vi "startAD.vi"() -> ()   [LabVIEW 2018]
uses:
  main/PCI8552B_32.dll
panel:
  out "待读取数据长度":i32
  out "波形图":dbl[][](graph)
  out "Data":dbl[][](array[numeric])
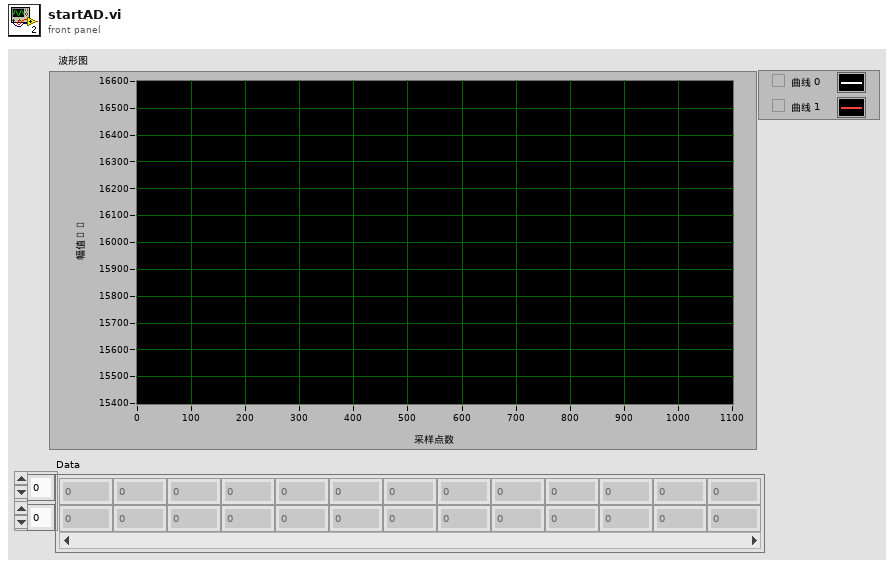
[diagram p1: front panel]
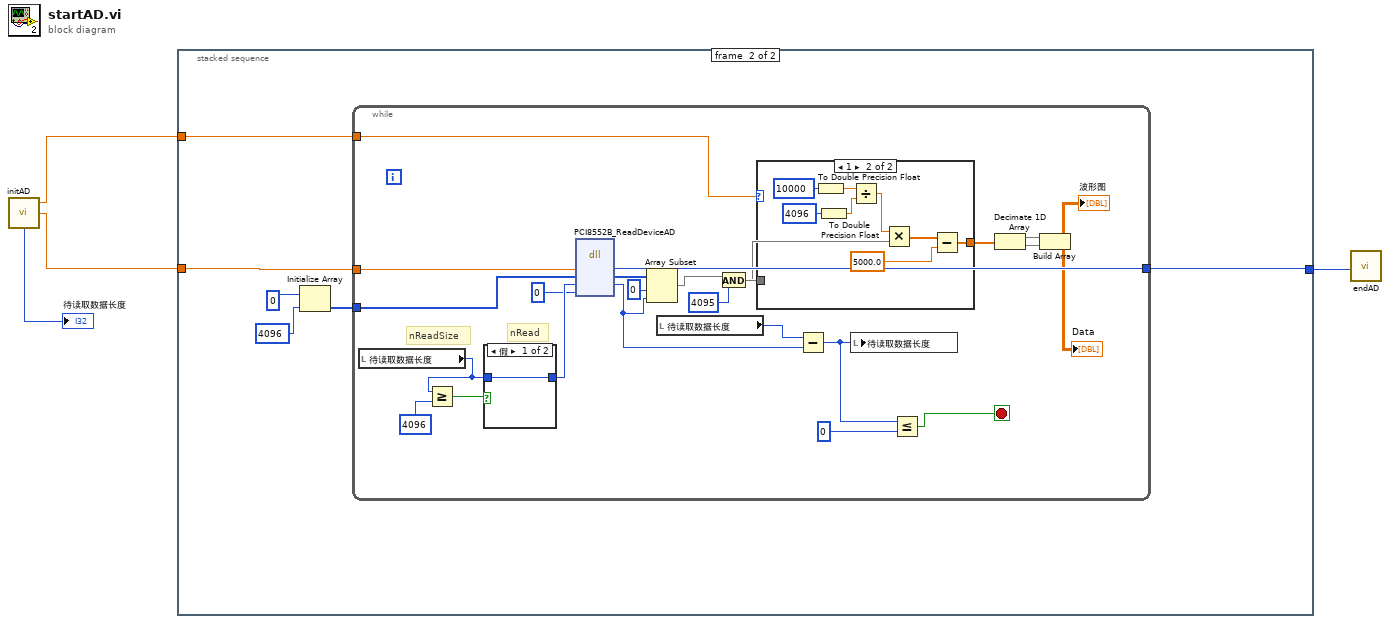
[diagram p0: block diagram]
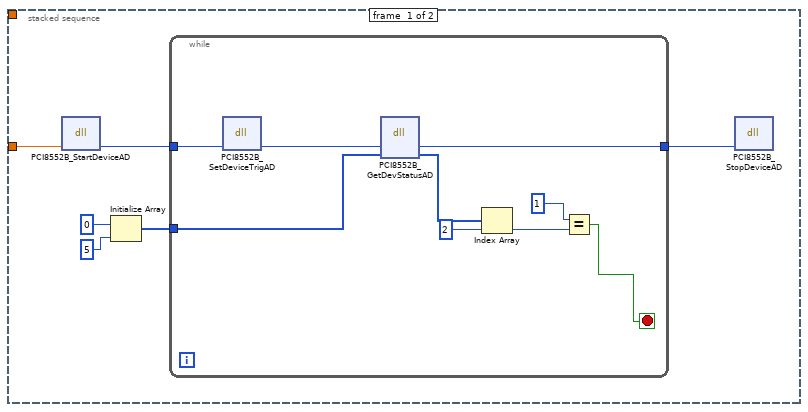
[diagram p2: hidden frame]
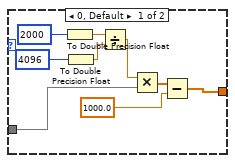
[diagram p3: hidden frame]
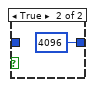
[diagram p4: hidden frame]
diagram:
  n1 = call "initAD.vi"() -> ("待读取数据长度"=→"待读取数据长度":i32, "采样频率"=w4:dbl, "设备"=w3:dbl)
  n2 = stacked-sequence {
    tunnel: w4 -> [w6 w21]
    tunnel: [_ w25] -> w1
    tunnel: w3 -> [_ w20]
    frame #0 {
      n3 = dll-call lib="PTH2…abs E\nPersonal Fileç ”ç©¶ç”Ÿå­¦ä¹ 202002-202007ç ”ä¸€ä¸‹å­¦æœŸwork2020\nSARControllerSAR-ControllermainPCI8552B_32.DLL" fn="PCI8552B_StartDeviceAD" label="StartDeviceAD"("hDevice"=w6) -> ("hDevice"=w5:i32)  [unwired: 4 in, 2 out]
      n4 = Initialize Array(0, 5) -> (w10:i32[])
      n5 = while {
        tunnel: w5 -> [w14]
        tunnel: w10 -> [w19]
        tunnel: [w12] -> w7
        stop <- w11 stop-if-true
        n6 = dll-call lib="PTH2…abs E\nPersonal Fileç ”ç©¶ç”Ÿå­¦ä¹ 202002-202007ç ”ä¸€ä¸‹å­¦æœŸwork2020\nSARControllerSAR-ControllermainPCI8552B_32.DLL" fn="PCI8552B_SetDeviceTrigAD" label="SetDeviceTrigAD"("hDevice"=w14) -> ("hDevice"=w13:i32)  [unwired: 4 in, 2 out]
        n7 = dll-call lib="PTH2…abs E\nPersonal Fileç ”ç©¶ç”Ÿå­¦ä¹ 202002-202007ç ”ä¸€ä¸‹å­¦æœŸwork2020\nSARControllerSAR-ControllermainPCI8552B_32.DLL" fn="PCI8552B_GetDevStatusAD" label="GetDevStatusAD"("hDevice"=w13, "ADStatus"=w19) -> ("hDevice"=w12:i32, "ADStatus"=w15:i32[])  [unwired: 4 in, 2 out]
        n8 = Index Array(array=w15, index=2) -> (element=w17:i32)
        n9 = Equal?(x=1, y=w17) -> (x = y?=w11:bool)
      }
      n10 = dll-call lib="PTH2…abs E\nPersonal Fileç ”ç©¶ç”Ÿå­¦ä¹ 202002-202007ç ”ä¸€ä¸‹å­¦æœŸwork2020\nSARControllerSAR-ControllermainPCI8552B_32.DLL" fn="PCI8552B_StopDeviceAD" label="StopDeviceAD"("hDevice"=w7) -> ()  [unwired: 5 in, 2 out]
    }
    frame #1 {
      n11 = Initialize Array(u16 0 ("y"), 4096 ("y")) -> (w22:u16[])
      n12 = while {
        tunnel: w21 -> [w48]
        tunnel: [w47] -> w25
        tunnel: w22 -> [w46]
        tunnel: w20 -> [w36]
        stop <- w26 stop-if-true
        # "nReadSize"
        # "nRead"
        n13 = local read "待读取数据长度"() -> (w42:i32)
        n14 = Greater Or Equal?(x=w42, y=4096 ("millisecond multiple")) -> (x >= y?=w44:bool)
        n15 = case shown="假" w44 {
          tunnel: [w67 4096 ("millisecond multiple")] -> w39
          tunnel: w42 -> [w67 _]
          frame False {
          }
          frame True {
          }
        }
        n16 = dll-call lib="PTH2…abs E\nPersonal Fileç ”ç©¶ç”Ÿå­¦ä¹ 202002-202007ç ”ä¸€ä¸‹å­¦æœŸwork2020\nSARControllerSAR-ControllermainPCI8552B_32.DLL" fn="PCI8552B_ReadDeviceAD" label="ReadDeviceAD"("hDevice"=w48, "pADBuffer"=w46, "nReadSizeWords"=w39, "nRetSizeWords"=0) -> ("hDevice"=w47:i32, "pADBuffer"=w33:u16[], "nReadSizeWords"=w30:u32)  [unwired: 5 in, 2 out]
        n17 = Array Subset(array=w33, index=0 ("索引"), length=w30) -> (w32:u16[])
        n18 = local read "待读取数据长度"() -> (w41:i32)
        n19 = And(x=w32, y=u16 4095) -> (x .and. y?=w37:u16[])
        n20 = case shown="1" w36 {
          tunnel: w37 -> [w56 w61]
          tunnel: [w49 w60] -> w35
          frame 0, Default {
            n21 = To Double Precision Float(number=2000 ("x")) -> (double precision float=w52:dbl)
            n22 = To Double Precision Float(number=4096) -> (double precision float=w51:dbl)
            n23 = Divide(x=w52, y=w51) -> (x/y=w57:dbl)
            n24 = Multiply(x=w57, y=w56) -> (x*y=w55:dbl[])
            n25 = Subtract(x=w55, y=1000.0) -> (x-y=w49:dbl[])
          }
          frame 1 {
            n26 = To Double Precision Float(number=10000 ("x")) -> (double precision float=w59:dbl)
            n27 = To Double Precision Float(number=4096) -> (double precision float=w63:dbl)
            n28 = Divide(x=w59, y=w63) -> (x/y=w66:dbl)
            n29 = Multiply(x=w66, y=w61) -> (x*y=w65:dbl[])
            n30 = Subtract(x=w65, y=5000.0) -> (x-y=w60:dbl[])
          }
        }
        n31 = Subtract(x=w41, y=w30) -> (x-y=w40:u32)
        n32 = local write "待读取数据长度"(w40) -> ()
        n33 = Less Or Equal?(x=w40, y=0) -> (x <= y?=w26:bool)
        n34 = Decimate 1D Array(w35) -> (w29:dbl[], w28:dbl[])
        n35 = Build Array(w29, w28) -> (→"波形图" →"Data":dbl[][])
      }
    }
  }
  n36 = call "endAD.vi"("设备"=w1) -> ()
